vi "GetDiagramInputs.vi"(6 "error in":errorcluster, 9 "DiagramDisable in":refnum<class "DiagramDisable.lvclass">) -> (0 "error out":errorcluster, 3 "DiagramDisable out":refnum<class "DiagramDisable.lvclass">, 4 "inputs terminals":refnum<class "Terminal.lvclass">[][](array[class]))   [LabVIEW 2014, in "DiagramDisable.lvclass"]
uses:
  DiagramDisable.lvclass
  Terminal/Terminal.lvclass
  DiagramDisable.lvclass/DiagramDisable.ctl
  Structure/Structure.lvclass
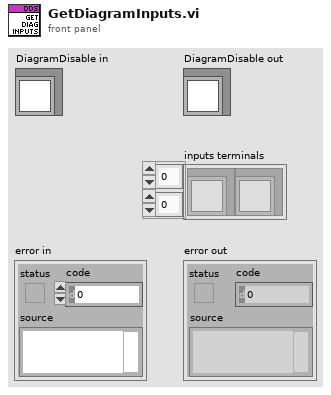
[diagram p1: front panel]
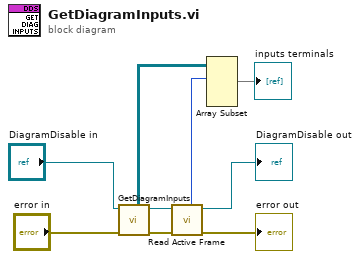
[diagram p0: block diagram]
diagram:
  n1 = call-parent "GetDiagramInputs.vi"("error in"="error in", "Structure in"="DiagramDisable in") -> ("error out"=→"error out":errorcluster, "Structure out"=w6:refnum<class "DiagramDisable.lvclass">, "inputs terminals"=w3:refnum<class "Terminal.lvclass">[][])  [unwired: 5 in]
  n2 = call "Read Active Frame.vi"("DiagramDisable in"=w6) -> ("DiagramDisable out"=→"DiagramDisable out":refnum<class "DiagramDisable.lvclass">, "Active Frame"=w1:i16)  [unwired: 7 in]
  n3 = Array Subset(array=w3, index (row)=w1) -> (→"inputs terminals":refnum<class "Terminal.lvclass">[][])  [unwired: 3 in]
